vi "StopImageAcquisition.vi"(8 "error in (no error)":errorcluster, 11 "Communication in":refnum<class "Microscope.lvclass">) -> (0 "error out":errorcluster, 3 "Communication out":refnum<class "Microscope.lvclass">)   [LabVIEW 2020, in "Microscope.lvlib" / "Microscope.lvclass"]
uses:
  Microscope.lvclass
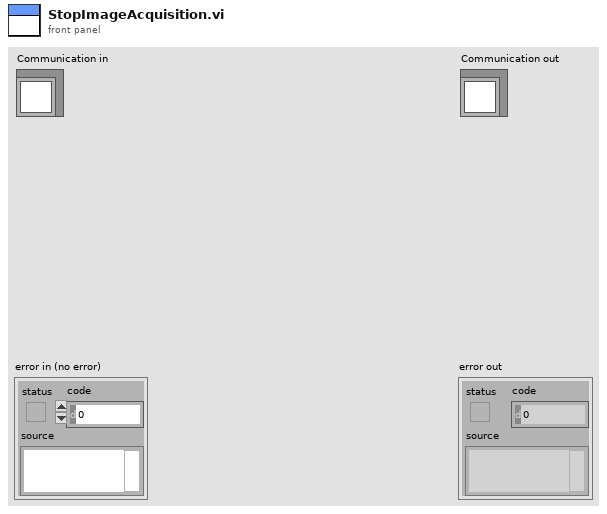
[diagram p1: front panel]
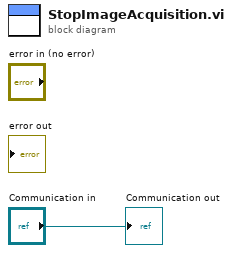
[diagram p0: block diagram]
diagram:
  "Communication out" <- "Communication in"
